vi "Get_Folders_on_Server.vi"(0 "Relative Path":path) -> (1 "Folder Names":string[](array[string]), 3 "error out":errorcluster)   [LabVIEW 2011]
uses:
  Anemometry/Anemometry Sub Vis/Globals/Constants_global.vi
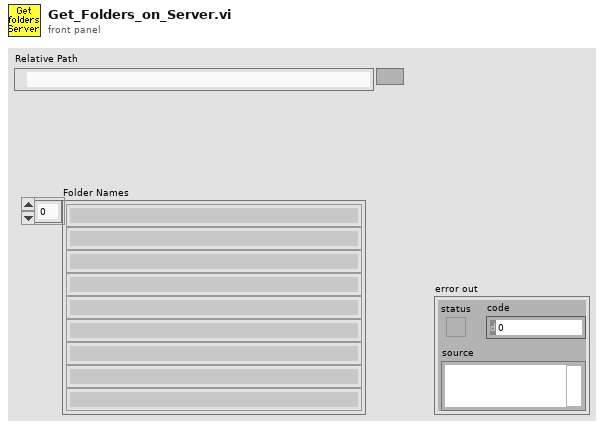
[diagram p1: front panel]
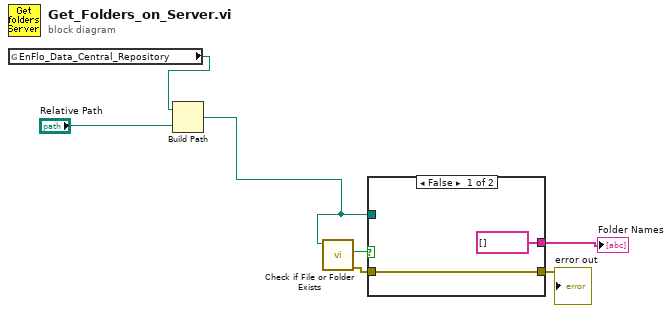
[diagram p0: block diagram]
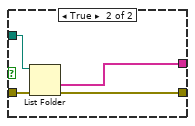
[diagram p2: hidden frame]
diagram:
  n1 = global read "Constants_global.vi" "EnFlo_Data_Central_Repository"() -> (w7:path)
  n2 = Build Path(base path=w7, name or relative path="Relative Path") -> (appended path=w5:path)
  n3 = call <vilib>:"Check if File or Folder Exists.vi"("path"=w5) -> ("error out"=w2:errorcluster, "file or folder exists?"=w6:bool)  [unwired: 8 in, 1 out]
  n4 = case shown="False" w6 {
    tunnel: [string[] [] ("folder names") w12] -> w4
    tunnel: w5 -> [_ w13]
    tunnel: w2 -> [w8 w11]
    tunnel: [w8 w10] -> w1
    frame False {
    }
    frame True {
      n5 = List Folder(path=w13, error in=w11) -> (folder names=w12:string[], error out=w10:errorcluster)  [unwired: 2 in, 2 out]
    }
  }
  "Folder Names" <- w4
  "error out" <- w1
